vi "ADC_GetConfig LVlink.vi"(7 "DeviceIndex":u32, 8 "error in (no error)":errorcluster) -> (0 "error out":errorcluster, 1 "End Channel":u8 format="%.0x", 2 "Start Channel":u8 format="%.0x", 3 "Channels":T3, 4 "Oversamples":u8, 5 "Calibration Mode":T2, 6 "Trigger & Counter bits":T1)   [LabVIEW 8.6]
doc: "Calls the ADC_GetConfig function and formats the data to give:\nChannel Info\nCalibration Mode\nTrigger & Counter Bits\nEnd Channel\nStart Channel\nOversamples"
uses:
  Controls/Gain Mode.ctl
  Controls/ADC_Setconfig.ctl
  Controls/Calibration Mode.ctl
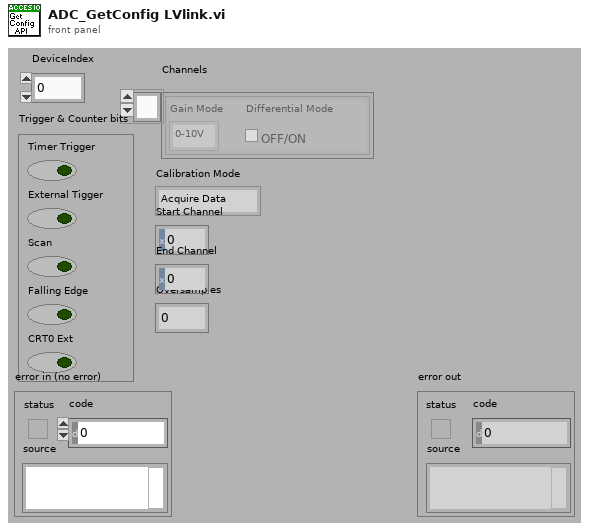
[diagram p1: front panel]
types:
  T1 = cluster{"Timer Trigger":bool, "External Tigger":bool, "Scan":bool, "Falling Edge":bool, "CRT0 Ext":bool}
  T2 = typedef "Calibration Mode.ctl" = enum8{"Acquire Data", "Acquire Ground", "Do not use", "Aquire Cal. Ref."}
  T3 = typedef "ADC_Setconfig.ctl" = cluster{"Gain Mode":T4, "Differential Mode":bool}[]
  T4 = typedef "Gain Mode.ctl" = enum8{"0-10V", "+/- 10V", "0-5V", "+/- 5V", "0-2V", "+/- 2V", "0-1V", "+/- 1V"}
  T5 = cluster{"Boolean array[0]":bool, "Boolean array[1]":bool, "Boolean array[2]":bool, "Boolean array[3]":bool, "Boolean array[4]":bool}
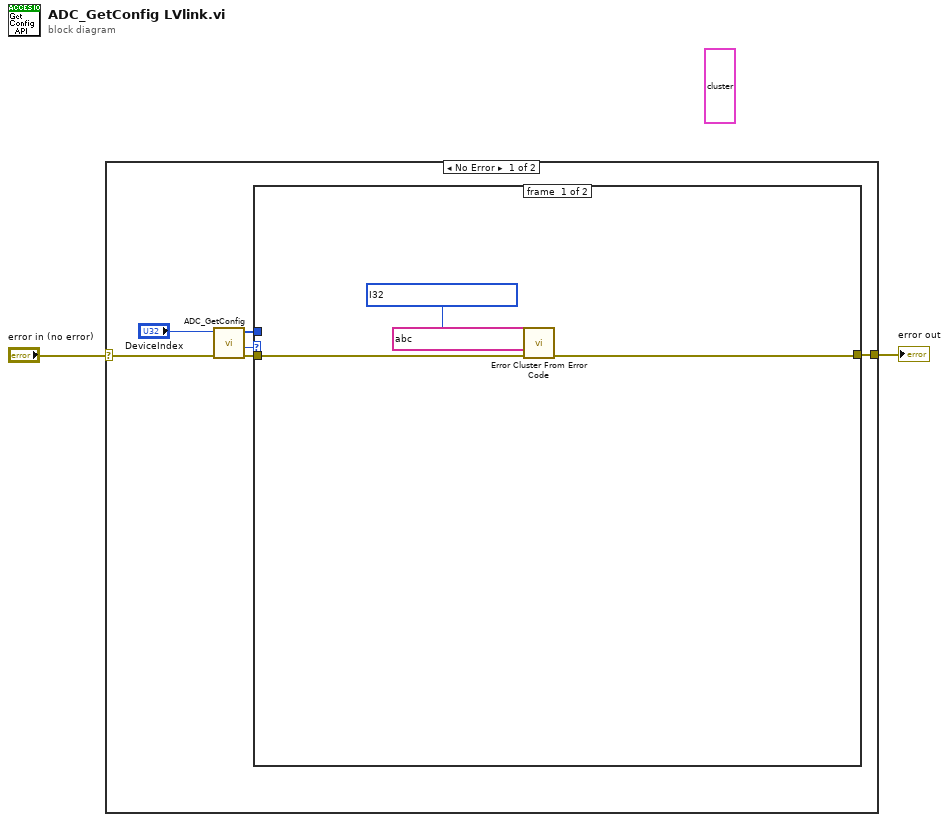
[diagram p0: block diagram]
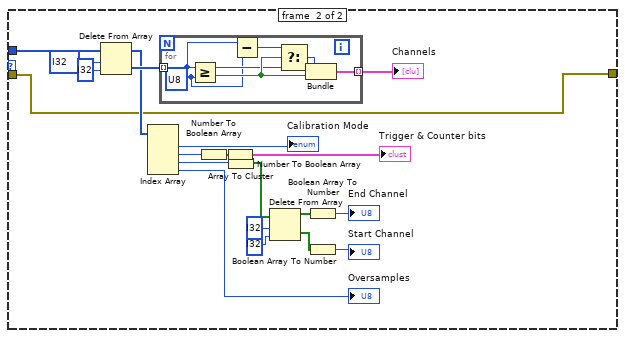
[diagram p2: hidden frame]
diagram:
  (unwired) T1 ? ("Trigger & Counter bits 2")
  n1 = case shown="No Error" "error in (no error)" {
    selector: "error in (no error)" -> [w8 w39]
    tunnel: [w5 w39] -> w2
    frame #0 {
      n2 = call "ADC_GetConfig.vi"("error in (no error)"=w8, "DeviceIndex"="DeviceIndex") -> ("error out"=w7:errorcluster, "ConfigBufSize"=w4:u32, "pConfigBuf"=w3:u8[])  [unwired: 7 in]
      n3 = case shown="20" w4 {
        tunnel: w7 -> [w12 w22]
        tunnel: [w11 w22] -> w5
        tunnel: w3 -> [_ w25]
        frame #0 {
          w10 = i32 ? items=["No error", "Argument error", "Memory is full", "Out of zone", "End of file", "File already open", "Generic file I/O error", "File not found", "File permission error", "Disk is full", "Duplicate path", "Too many files open", "System feature not enabled", "Resource file not found", "Cannot add resource", "Resource not found", "Image not found", "Image memory error", "Pen does not exist", "Config type invalid", "Config token not found", "Config parse error", "Config memory error", "Bad external code format", "Bad external code offset", "External code not present", "Null window", "Destroy window error", "Null menu", "Print aborted", "Bad print record", "Print driver error", "Windows error during printing", "Memory error during printing", "Print dialog error", "Generic print error", "Invalid device refnum", "Device not found", "Device parameter error", "Device unit error", "Cannot open device", "Device call aborted", "Generic error", "Cancelled by user", "Object ID too low", "Object ID too high", "Object not in heap", "Unknown heap", "Unknown object (invalid DefProc)", "Unknown object (DefProc not in table)", "Message out of range", "Invalid (null) method", "Unknown message", "Manager call not supported", "Bad address", "Network operation in progress", "Network operation timed out", "Connection is busy", "Network attribute not supported", "Network error", "Address in use", "System out of memory", "Connection aborted", "Connection refused", "Not connected", "Already connected", "Connection closed", "Initialization error (interapplication manager)", "Bad occurrence", "Wait on unbound occurrence handler", "Occurrence queue overflow", "Datalog type conflict", "Unused", "Unrecognized type (interapplication manager)", "Memory corrupt", "Failed to make temporary DLL", "Old CIN version", "Drag socket not found", "Failed to load drop-object", "Failed to register OLE object", "Failed to release OLE object", "Format specifier type mismatch", "Unknown format specifier", "Too few format specifiers", "Too many format specifiers", "Scan failed", "Newer CIN version", "Error converting to variant", "Runtime menu error", "Password tampered", "Variant attribute not found", "Incompatible variant data type", "Event data is not available", "Event Store is not present", "Occurrence is not found", "Event Queue is not created", "Event info is not available", "Refnum passed is NULL", "Error retrieving Class GUID", "Error retrieving CoClass GUID", "Error retrieving TypeLib GUID.", "Bad built application magic bytes.", "Specific driver is different from the specific driver associated with the Logical Name.", "There is no session opened to the class driver.", "Max Error", "MAX - Error with config objects", "MAX - Error loading configuration", "MAX - Group not supported"]
          n4 = call <vilib>:"Error Cluster From Error Code.vi"("error in (no error)"=w12, "error message (\"\")"=string ? ("error message (\"\")"), "error code (0)"=w10) -> ("error out"=w11:errorcluster)  [unwired: 6 in]
        }
        frame #1 {
          n5 = Delete From Array(array=w25, length=i32 ?, index=i32 ?) -> (deleted portion=w30:u8[], array with subset deleted=w29:u8[])
          n6 = Index Array(array=w29) -> (element #1=→"Calibration Mode":u8, element #2=w27:u8, element #3=w13:u8, element #4=→"Oversamples":u8)  [unwired: 4 in]
          n7 = for {
            tunnel: w30 -> [w34] mode=indexing
            tunnel: [w38] -> w32 mode=indexing
            w33 = u8 ?
            n8 = Greater Or Equal?(x=w34, y=w33) -> (x >= y?=w36:bool)
            n9 = Subtract(x=w34, y=w33) -> (x-y=w35:u8)
            n10 = Select(t=w35, s=w36, f=w34) -> (s? t:f=w37:u8)
            n11 = Bundle(w37, w36) -> (w38:cluster{u8, bool})  [unwired: 1 in]
          }
          "Channels" <- w32
          n12 = Number To Boolean Array(number=w27) -> (Boolean array=w28:bool[])
          n13 = Array To Cluster(array=w28) -> (cluster=→"Trigger & Counter bits":T5)
          n14 = Number To Boolean Array(number=w13) -> (Boolean array=w16:bool[])
          n15 = Delete From Array(array=w16, length=i32 ? ("index"), index=i32 ? ("length")) -> (deleted portion=w18:bool[], array with subset deleted=w17:bool[])
          n16 = Boolean Array To Number(Boolean array=w17) -> (number=→"End Channel":u32)
          n17 = Boolean Array To Number(Boolean array=w18) -> (number=→"Start Channel":u32)
        }
      }
    }
    frame #1 {
    }
  }
  "error out" <- w2
